vi "AFT Filter Signal and Update Coefficients.vi"   [LabVIEW 2017, in "NI_AdaptiveFilter.lvlib"]
doc: "Filters an input signal with an adaptive filter and updates the coefficients of the adaptive filter iteratively. You must use the least mean squares (LMS) or recursive least squares (RLS) algorithms to create the adaptive filter. Wire data to the <B>x(n)</B> and <B>d(n)</B> inputs to determine the polymorphic instance to use or manually select the instance. The data type of the adaptive filter that you wire to the <B>adaptive filter in</B> input must match the instance of the AFT Filter Signal and Update Coefficients VI."
uses:
  <vilib>/addons/Adaptive Filters/NI_AdaptiveFilter.lvlib
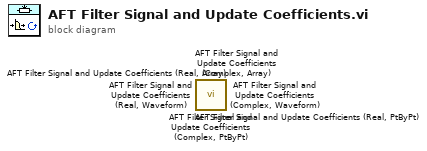
[diagram p0: block diagram]
diagram:
  n1 = call <vilib>:"AFT Filter Signal and Update Coefficients (Complex, PtByPt).vi"() -> ()  [unwired: 8 in, 4 out]
  n2 = call <vilib>:"AFT Filter Signal and Update Coefficients (Complex, Array).vi"() -> ()  [unwired: 8 in, 4 out]
  n3 = call <vilib>:"AFT Filter Signal and Update Coefficients (Real, Waveform).vi"() -> ()  [unwired: 8 in, 4 out]
  n4 = call <vilib>:"AFT Filter Signal and Update Coefficients (Complex, Waveform).vi"() -> ()  [unwired: 8 in, 4 out]
  n5 = call <vilib>:"AFT Filter Signal and Update Coefficients (Real, Array).vi"() -> ()  [unwired: 8 in, 4 out]
  n6 = call <vilib>:"AFT Filter Signal and Update Coefficients (Real, PtByPt).vi"() -> ()  [unwired: 8 in, 4 out]
